vi "TCP Listen Internal List.vi"(8 "Index #":i32, 9 "Element In":cluster{u16, refnum<k5>}, 10 "Port":u16, 11 "Operation":T1) -> (0 "Element # \n(-1 if not found)":i32, 3 "Item Requested":cluster{u16, refnum<k5>})   [LabVIEW 2011]
uses:
  TCP Listen List Operations.ctl
panel:
  in  "Empty Element":cluster{u16, refnum<k5>}
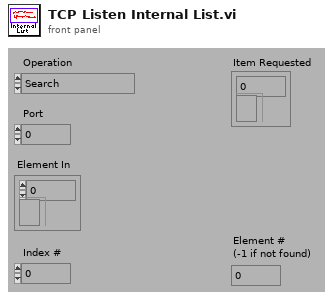
[diagram p1: front panel]
types:
  T1 = typedef "TCP Listen List Operations.ctl" = enum16{"Search", "Retrieve Element", "Add Element", "Delete Element"}
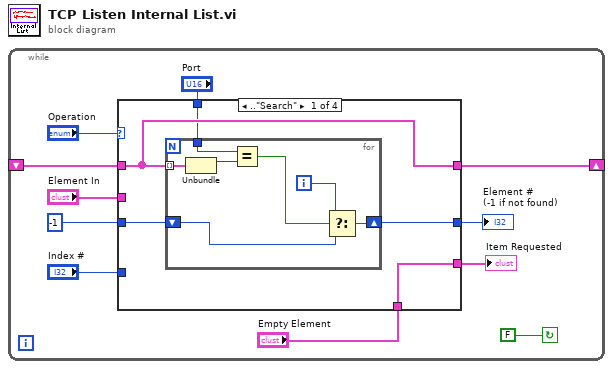
[diagram p0: block diagram]
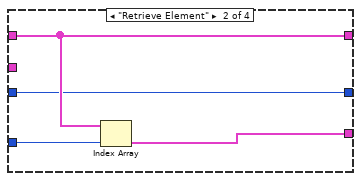
[diagram p2: hidden frame]
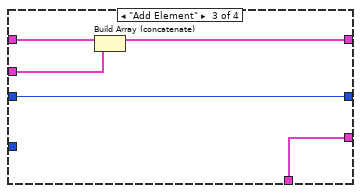
[diagram p3: hidden frame]
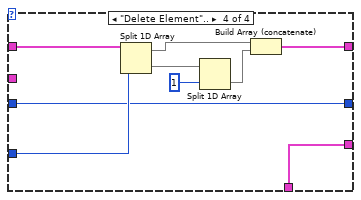
[diagram p4: hidden frame]
diagram:
  n1 = while {
    shift-left: _ -> [w9]
    shift-right: [w7] -> _
    stop <- FALSE continue-if-true
    n2 = case shown="..\"Search\"" "Operation" {
      tunnel: "Element In" -> [_ _ w31 _]
      tunnel: "Index #" -> [_ w27 _ w41]
      tunnel: w9 -> [w16 w26 w32 w40]
      tunnel: "Port" -> [w15 _ _ _]
      tunnel: [w16 w26 w30 w35] -> w7
      tunnel: [w14 w25 w29 w34] -> w5
      tunnel: -1 -> [w13 w25 w29 w34]
      tunnel: [w12 w24 w28 w33] -> w3
      tunnel: "Empty Element" -> [w12 _ w28 w33]
      frame .."Search" {
        n3 = for {
          tunnel: w16 -> [w23] mode=indexing
          tunnel: w15 -> [w22]
          shift-right: [w17] -> w14
          shift-left: w13 -> [w19]
          i -> [w20]
          n4 = Unbundle(w23) -> (w21:u16)  [unwired: 1 out]
          n5 = Equal?(x=w22, y=w21) -> (x = y?=w18:bool)
          n6 = Select(t=w20, s=w18, f=w19) -> (s? t:f=w17:i32)
        }
      }
      frame "Retrieve Element" {
        n7 = Index Array(array=w26, index=w27) -> (element=w24:cluster{u16, refnum<k5>})
      }
      frame "Add Element" {
        n8 = Build Array (concatenate)(w32, w31) -> (w30:cluster{u16, refnum<k5>}[])
      }
      frame "Delete Element".. {
        n9 = Split 1D Array(array=w40, index=w41) -> (first subarray=w36:cluster{u16, refnum<k5>}[], second subarray=w38:cluster{u16, refnum<k5>}[])
        n10 = Split 1D Array(array=w38, index=1) -> (second subarray=w37:cluster{u16, refnum<k5>}[])  [unwired: 1 out]
        n11 = Build Array (concatenate)(w36, w37) -> (w35:cluster{u16, refnum<k5>}[])
      }
    }
    "Element # \n(-1 if not found)" <- w5
    "Item Requested" <- w3
  }
